vi "Dresser DXD Reset.vi"(0 "VISA session":refnum<visa-resource-name>, 5 "DXD Address (1)":T1=1 min=1 max=99 step=1, 11 "Error In (no error)":errorcluster) -> (4 "dup VISA session":refnum<visa-resource-name>, 15 "Error Out":errorcluster)   [LabVIEW 2015]
doc: "CAUTION: Using this VI may be hazardous to the functionality of the Dresser DXD Series pressure transducer. A zero is written to all unlocked locations in the EEPROM.\n\nThis VI resets the Dresser DXD Series pressure transducer by initializing the EEPROM with the 'ez' command, and then sends a set of default setup commands to the instrument.\n\nWritten by:\nBLOOMY CONTROLS, INC\nWINDSOR, CT 06095, USA\n860-298-9925\nwww.bloomy.com\nV2.0.0\nMay, 2002"
uses:
  Type Defs/DXD Address.ctl
panel:
  # "For instructions on the use of this VI, press Ctrl+H to display the help window and move the mouse over the icon, controls, and indicators"
  # "CAUTION: Using this VI may be\nhazardous to the functionality of\nthe Dresser DXD Series pressure\ntransducer.  A zero is written to all\nunlocked locations in the EEPROM"
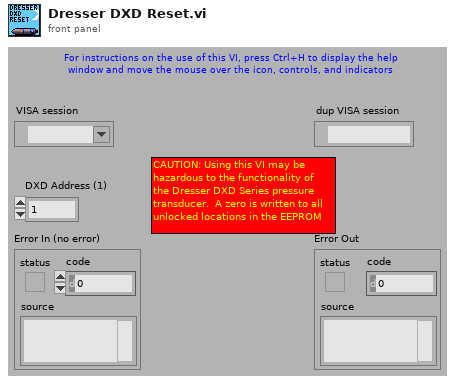
[diagram p1: front panel]
types:
  T1 = typedef "DXD Address.ctl" = i32
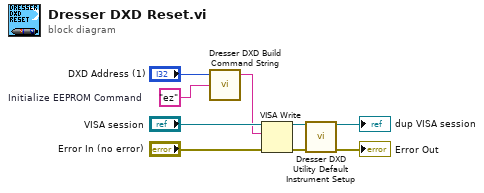
[diagram p0: block diagram]
diagram:
  w2 = "ez"  # Initialize EEPROM Command
  n1 = call "Dresser DXD Build Command String.vi"("Command Mnemonic (\"\")"=w2, "DXD Address (1)"="DXD Address (1)") -> ("Command String"=w1:string)  [unwired: 3 in]
  n2 = VISA Write(VISA resource name="VISA session", write buffer=w1, error in (no error)="Error In (no error)") -> (VISA resource name out=w4:refnum<visa-resource-name>, error out=w5:errorcluster)  [unwired: 1 out]
  n3 = call "Dresser DXD Utility Default Instrument Setup.vi"("VISA session"=w4, "Error In (no error)"=w5) -> ("dup VISA session"=→"dup VISA session":refnum<visa-resource-name>, "Error Out"=→"Error Out":errorcluster)  [unwired: 12 in]
